vi "Arm.vi"(8 "error in (no error)":errorcluster, 10 "Arm":bool=TRUE, 11 "Mag Lab Root in":refnum<class "Mag Lab Root.lvclass">) -> (0 "error out":errorcluster, 3 "Mag Lab Root out":refnum<class "Mag Lab Root.lvclass">)   [LabVIEW 2015, in "Mag Lab Root.lvclass"]
uses:
  Mag Lab Root.lvclass
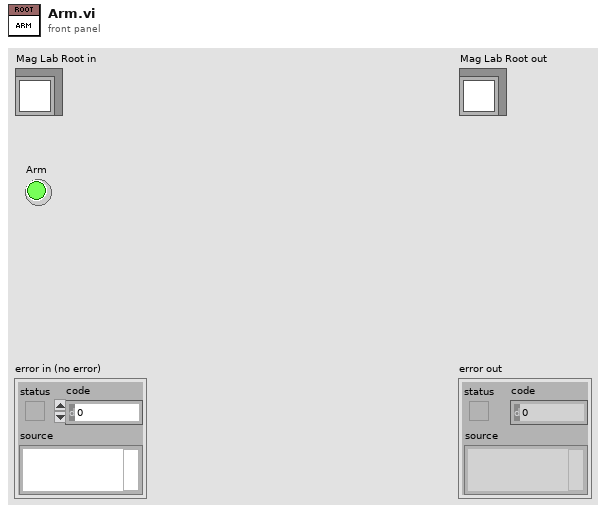
[diagram p1: front panel]
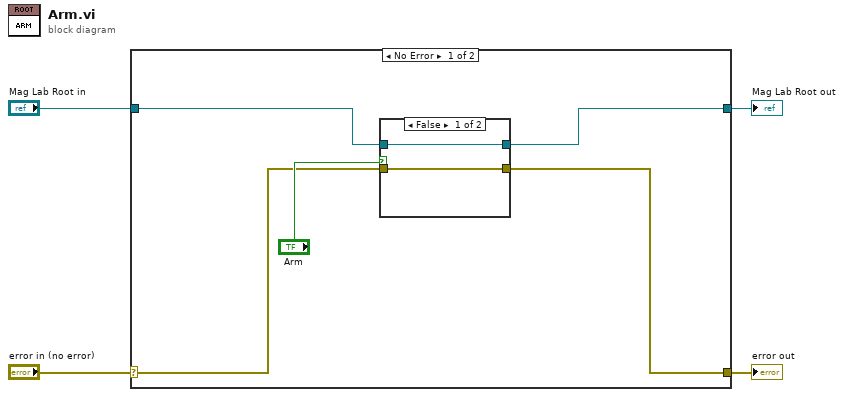
[diagram p0: block diagram]
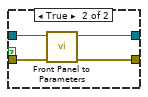
[diagram p2: hidden frame]
diagram:
  n1 = case shown="No Error" "error in (no error)" {
    selector: "error in (no error)" -> [w6 w17]
    tunnel: [w5 w17] -> w3
    tunnel: [w8 w16] -> w1
    tunnel: "Mag Lab Root in" -> [w9 w16]
    frame No Error {
      n2 = case shown="False" "Arm" {
        tunnel: w9 -> [w11 w15]
        tunnel: [w11 w14] -> w8
        tunnel: w6 -> [w10 w13]
        tunnel: [w10 w12] -> w5
        frame False {
        }
        frame True {
          n3 = call-dynamic "Front Panel to Parameters.vi"("error in (no error)"=w13, "Mag Lab Root in"=w15) -> ("error out"=w12:errorcluster, "Mag Lab Root out"=w14:refnum<class "Mag Lab Root.lvclass">)  [unwired: 8 in]
        }
      }
    }
    frame Error {
    }
  }
  "error out" <- w3
  "Mag Lab Root out" <- w1
